vi "Read Hardware Handles.vi"(8 "error in":errorcluster, 11 "Ballard ARINC-429 shared resources in":refnum<class "Ballard ARINC-429 Shared Resources.lvclass">) -> (0 "error out":errorcluster, 2 "hardware handles":T1, 3 "Ballard ARINC-429 shared resources out":refnum<class "Ballard ARINC-429 Shared Resources.lvclass">)   [LabVIEW 2020, in "Ballard ARINC 429 Engine.lvlib" / "Implementation.lvlib" / "Ballard ARINC-429 Shared Resources.lvclass"]
uses:
  Ballard ARINC-429 Shared Resources.lvclass
  Custom Device/Hardware Handles.ctl
  Ballard ARINC-429 Shared Resources.lvclass/Ballard ARINC-429 Shared Resources.ctl
  Custom Device/Custom Device.lvlib
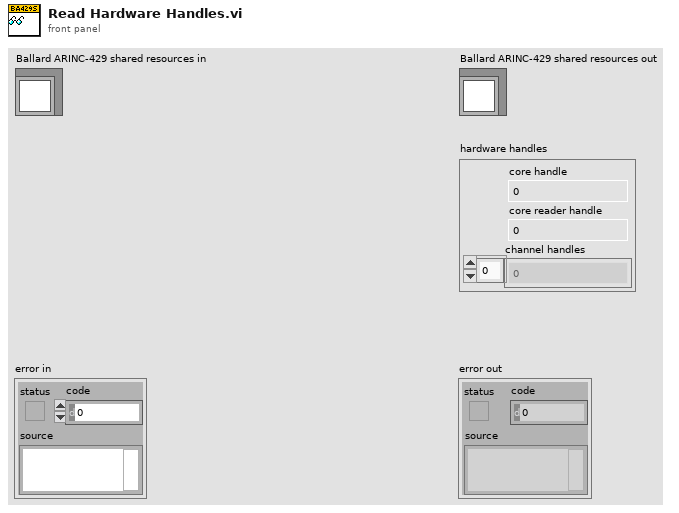
[diagram p1: front panel]
types:
  T1 = typedef "Ballard ARINC 429 Engine.lvlib/Custom Device.lvlib/Hardware Handles.ctl" = cluster{"core handle":u64, "core reader handle":u64, "channel handles":u64[]}
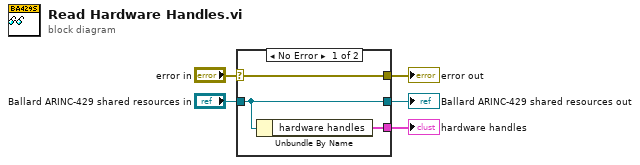
[diagram p0: block diagram]
diagram:
  n1 = case shown="No Error" "error in" {
    selector: "error in" -> [w8 w9]
    tunnel: [w8 w9] -> w4
    tunnel: [w7 w10] -> w2
    tunnel: "Ballard ARINC-429 shared resources in" -> [w7 w10]
    tunnel: [w6 _] -> w1
    frame No Error {
      n2 = Unbundle By Name(w7) -> ("hardware handles"=w6:T1)
    }
    frame Error {
    }
  }
  "error out" <- w4
  "Ballard ARINC-429 shared resources out" <- w2
  "hardware handles" <- w1
